vi "distance.vi"(10 "Goal \nplatform":i32, 11 "Start \nplatform":i32) -> (3 "distance":i32)   [LabVIEW 2017]
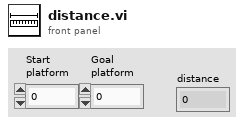
[diagram p1: front panel]
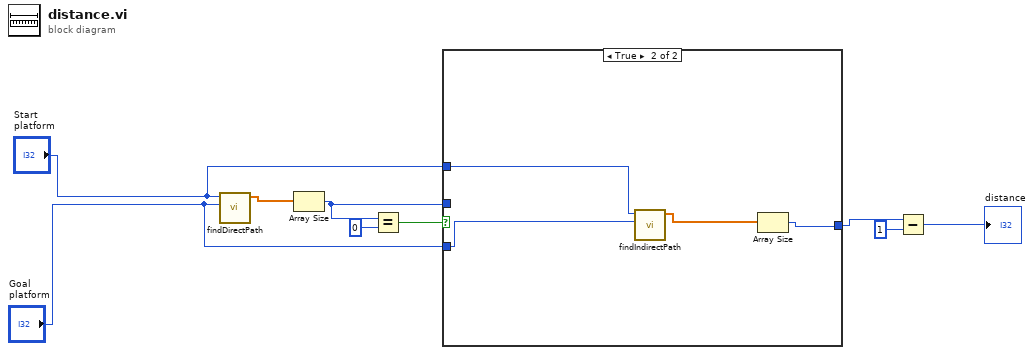
[diagram p0: block diagram]
diagram:
  n1 = call "findDirectPath.vi"("goal platform"="Goal \nplatform", "start platform"="Start \nplatform") -> ("path"=w9:dbl[])  [unwired: 6 in, 3 out]
  n2 = Array Size(array=w9) -> (size(s)=w4:i32)
  n3 = Equal?(x=w4, y=0) -> (x = y?=w7:bool)
  n4 = case shown="True" w7 {
    tunnel: "Start \nplatform" -> [_ w14]
    tunnel: "Goal \nplatform" -> [_ w13]
    tunnel: [w10 w11] -> w3
    tunnel: w4 -> [w10 _]
    frame False {
    }
    frame True {
      n5 = call "findIndirectPath.vi"("goal platform"=w13, "start platform"=w14) -> ("total path"=w12:dbl[])  [unwired: 4 in, 5 out]
      n6 = Array Size(array=w12) -> (size(s)=w11:i32)
    }
  }
  n7 = Subtract(x=w3, y=1) -> (x-y=→"distance":i32)
